vi "RTM - Add Tx Unbound Channels.vi"(8 "error in (no error)":errorcluster, 11 "Node Ptr":T1 format="%.0x") -> (0 "error out":errorcluster)   [LabVIEW 2019, in "UDP-Custom-Device System Explorer.lvlib"]
uses:
  UDP-Custom-Device System Explorer.lvlib
  <vilib>/NI VeriStand/Custom Device API/Custom Device Item Ref.ctl
  Shared/Types/Shared - Channel Data Type.ctl
  <vilib>/NI VeriStand/Custom Device API/Custom Device Channel.ctl
  <vilib>/NI VeriStand/Custom Device API/Custom Device Channel Type.ctl
  Shared/Constants.vi
  <vilib>/NI VeriStand/Custom Device API/Custom Device API.lvlib
  Shared/UDP-Custom-Device Shared.lvlib
  <vilib>/NI VeriStand/Custom Device Tools/Custom Device Utility Library/Custom Device Utility Library.lvlib
  Property Accessors/Tx Channel Accessors.lvlib
  Property Accessors/Tx Channel Section Accessors.lvlib
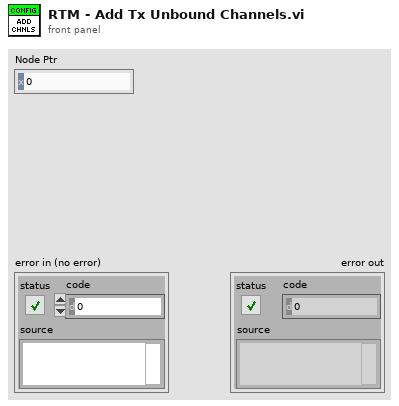
[diagram p1: front panel]
types:
  T1 = typedef "Custom Device API.lvlib/Custom Device Item Ref.ctl" = u64
  T2 = typedef "Custom Device API.lvlib/Custom Device Channel.ctl" = cluster{"Type":T3, "Units":string, "Default Value":dbl, "Faultable":bool, "Scalable":bool}
  T3 = typedef "Custom Device API.lvlib/Custom Device Channel Type.ctl" = enum16{"Input", "Output"}
  T4 = typedef "UDP-Custom-Device Shared.lvlib/Shared - Channel Data Type.ctl" = enum16{"Boolean", "Single", "Double", "I8", "I16", "I32", "I64", "U8", "U16", "U32", "U64"}
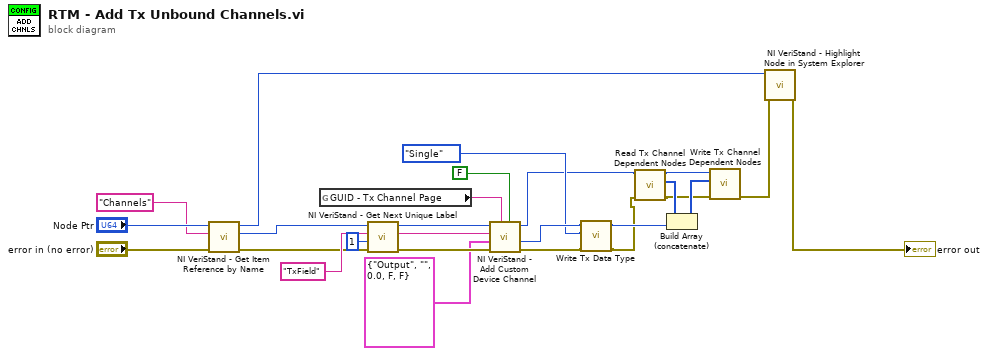
[diagram p0: block diagram]
diagram:
  n1 = call <vilib>:"NI VeriStand - Get Item Reference by Name.vi"("error in (no error)"="error in (no error)", "Item Name"="Channels" ("Section Name"), "Parent Ref in"="Node Ptr") -> ("error out"=w15:errorcluster, "Item Ref"=w14:T1, "Parent Ref out"=w13:T1)  [unwired: 5 in, 1 out]
  n2 = global read "Constants.vi" "GUID - Tx Channel Page"() -> (w26:string)
  n3 = call <vilib>:"NI VeriStand - Get Next Unique Label.vi"("error in (no error)"=w15, "Start Value (1)"=1, "Label"="TxField", "Parent Ref in"=w14) -> ("error out"=w23:errorcluster, "Label out"=w22:string, "Parent Ref dup"=w21:T1)  [unwired: 4 in, 1 out]
  n4 = call <vilib>:"NI VeriStand - Add Custom Device Channel.vi"("Highlight? (F)"=FALSE, "GUID (Default Channel)"=w26, "error in (no error)"=w23, "Channel"=T2 {"Type"=enum."Output", "Units"="", "Default Value"=0.0, "Faultable"=FALSE, "Scalable"=FALSE}, "Channel Name"=w22, "Parent Ref in"=w21) -> ("error out"=w9:errorcluster, "Channel Ref"=w11:T1, "Parent Ref out"=w7:T1)  [unwired: 2 in, 1 out]
  n5 = call "Write Tx Data Type.vi"("error in (no error)"=w9, "Data Type"=Shared_-_Channel_Data_Type."Single", "Node Ptr"=w11) -> ("error out"=w6:errorcluster, "Node Ptr out"=w8:T1)  [unwired: 7 in]
  n6 = call "Read Tx Channel Dependent Nodes.vi"("error in (no error)"=w6, "Node Ptr"=w7) -> ("error out"=w2:errorcluster, "Dependent Node Refs"=w5:T1[], "Node Ptr out"=w4:T1)  [unwired: 7 in]
  n7 = Build Array (concatenate)(w5, w8) -> (w3:T1[])
  n8 = call "Write Tx Channel Dependent Nodes.vi"("error in (no error)"=w2, "Dependent Node Refs"=w3, "Node Ptr"=w4) -> ("error out"=w1:errorcluster)  [unwired: 7 in, 1 out]
  n9 = call <vilib>:"NI VeriStand - Highlight Node in System Explorer.vi"("error in (no error)"=w1, "Item Ref in"=w13) -> ("error out"=→"error out":errorcluster)  [unwired: 8 in, 1 out]
